vi "Plot S-Curve.vi"() -> ()   [LabVIEW 2019]
uses:
  <vilib>/Analysis/NI_AALPro.lvlib
panel:
  out "x 3":dbl[](graph)
  out "v 3":dbl[](graph)
  out "x 2":dbl[](graph)
  out "v 2":dbl[](graph)
  in  "dt (s)":dbl=1.0
  in  "Limits":T1
  in  "goal":dbl
  out "a":dbl[](graph)
  out "x":dbl[](graph)
  out "v":dbl[](graph)
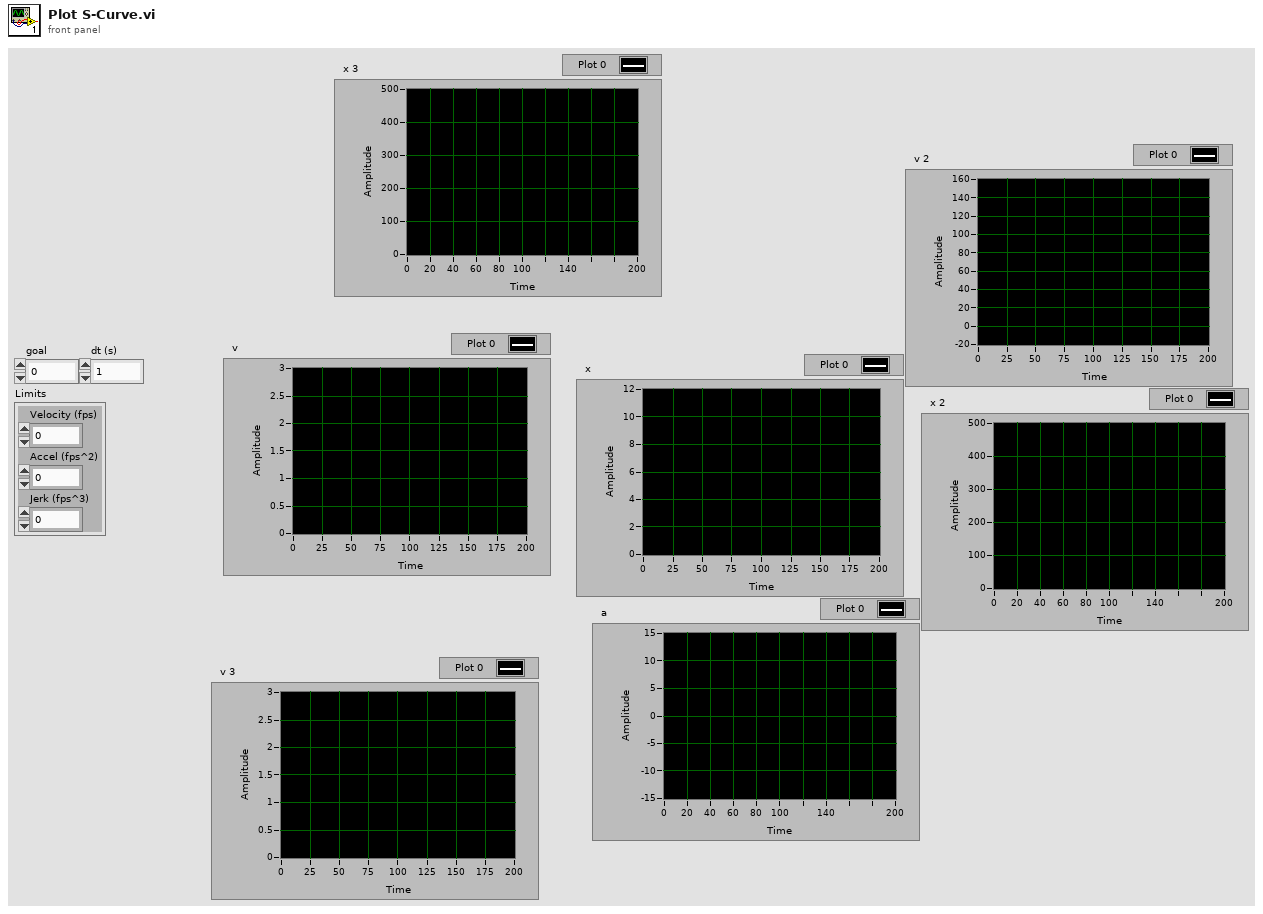
[diagram p1: front panel]
types:
  T1 = cluster{"Velocity (fps)":dbl, "Accel (fps^2)":dbl, "Jerk (fps^3)":dbl}
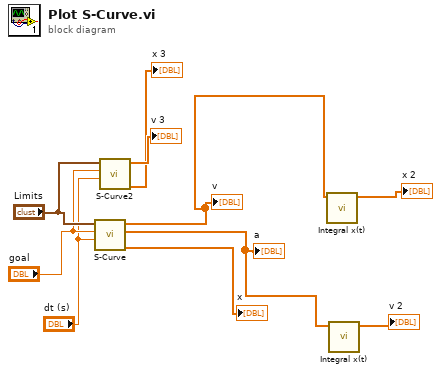
[diagram p0: block diagram]
diagram:
  n1 = call "S-Curve.vi"("dt (s)"="dt (s)", "goal"="goal", "Limits"="Limits") -> ("X"=→"x":dbl[], "A"=w9:dbl[], "V"=w7:dbl[])  [unwired: 5 in, 1 out]
  "v" <- w7
  "a" <- w9
  n2 = call "S-Curve2.vi"("dt (s)"="dt (s)", "goal"="goal", "Limits"="Limits") -> ("X"=→"x 3":dbl[], "V"=→"v 3":dbl[])  [unwired: 5 in, 2 out]
  n3 = call <vilib>:"Integral x(t).vi"("X"=w7) -> ("Integral X"=→"x 2":dbl[])  [unwired: 9 in, 1 out]
  n4 = call <vilib>:"Integral x(t).vi"("X"=w9) -> ("Integral X"=→"v 2":dbl[])  [unwired: 9 in, 1 out]
